vi "Read UDP Data.vi"(8 "error in (no error)":errorcluster, 11 "UDP Cluster in":T2) -> (0 "error out":errorcluster, 3 "UDP Cluster out":T2)   [LabVIEW 2013, in "Workspace MultiY Graph.lvlib"]
uses:
  Workspace MultiY Graph.lvlib
  UDP Stream Configuration.ctl
  <vilib>/NI Veristand/Execution/Workspace/UDP Stream Packet.ctl
  <vilib>/NI Veristand/Execution/Workspace/NI_VS Workspace ExecutionAPI.lvlib
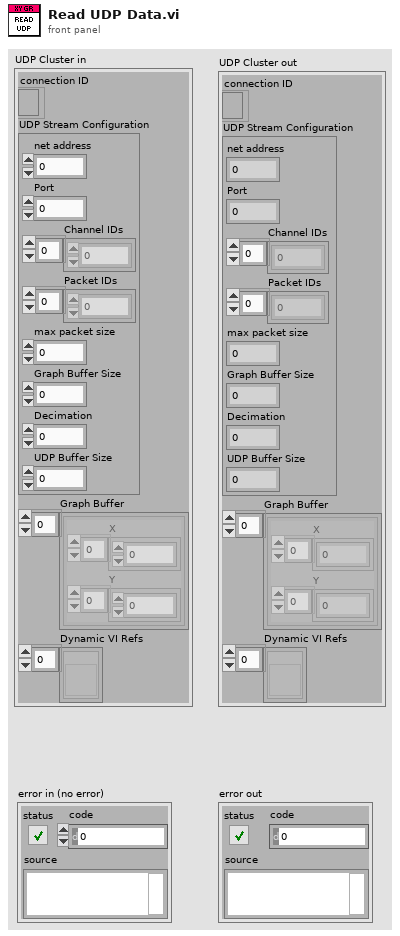
[diagram p1: front panel]
types:
  T1 = typedef "Workspace MultiY Graph.lvlib/UDP Stream Configuration.ctl" = cluster{"net address":u32, "Port":u16, "Channel IDs":i32[], "Packet IDs":i32[], "max packet size":i32, "Graph Buffer Size":i32, "Decimation":i32, "UDP Buffer Size":u32}
  T2 = cluster{"connection ID":refnum<k16>, "UDP Stream Configuration":T1, "Graph Buffer":cluster{"X":dbl[], "Y":dbl[]}[], "Dynamic VI Refs":refnum<vi>[]}
  T3 = typedef "NI_VS Workspace ExecutionAPI.lvlib/UDP Stream Packet.ctl" = cluster{"ID":i32, "t0":dbl, "dt":dbl, "Channel IDs":i32[], "Channel Data":dbl[][], "Sample Offset":u64}
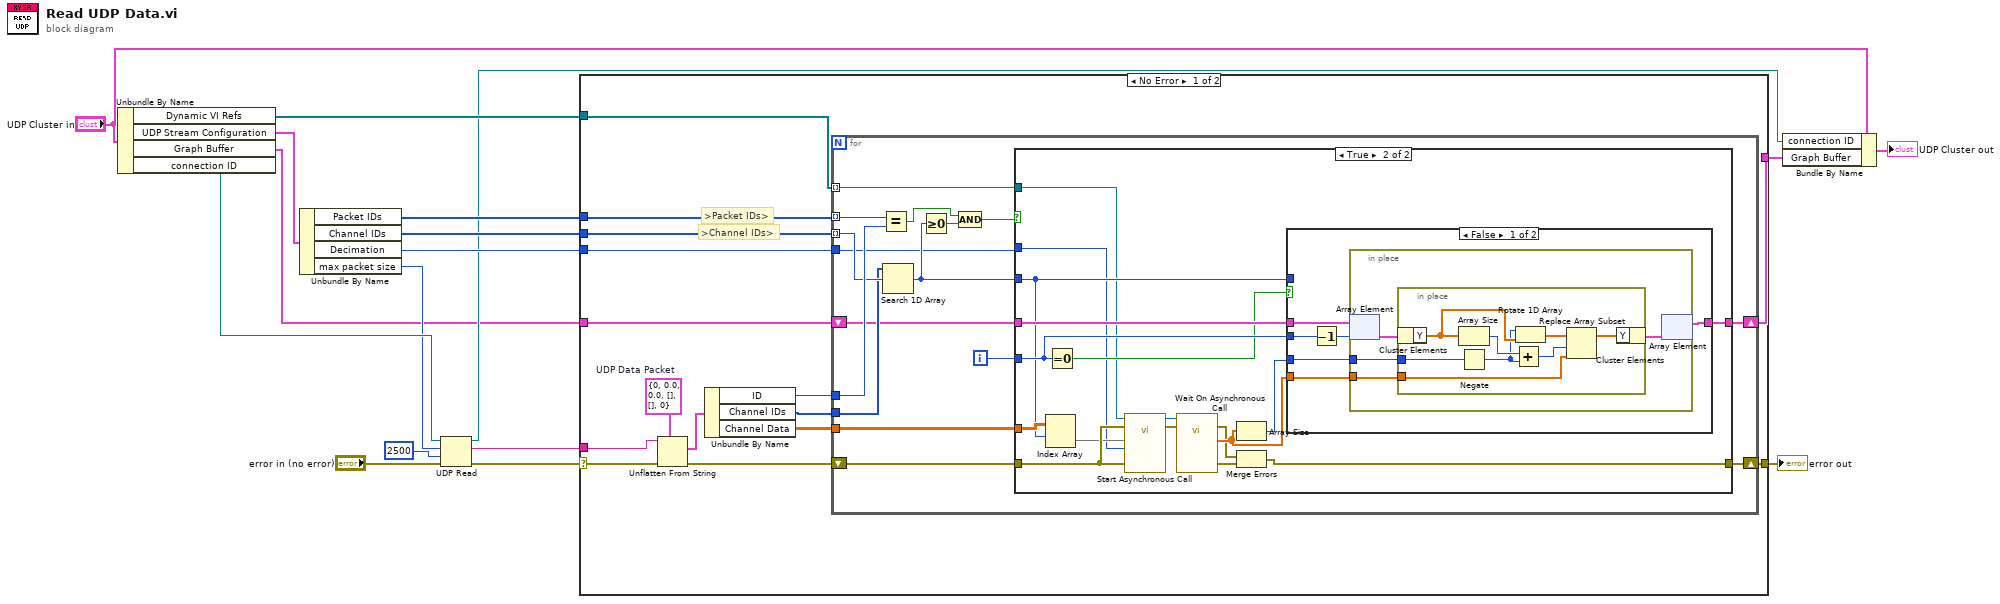
[diagram p0: block diagram]
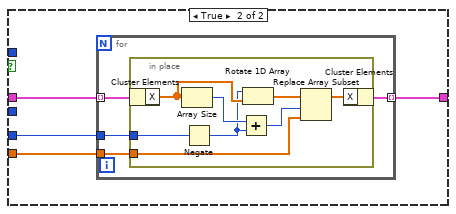
[diagram p3: hidden frame]
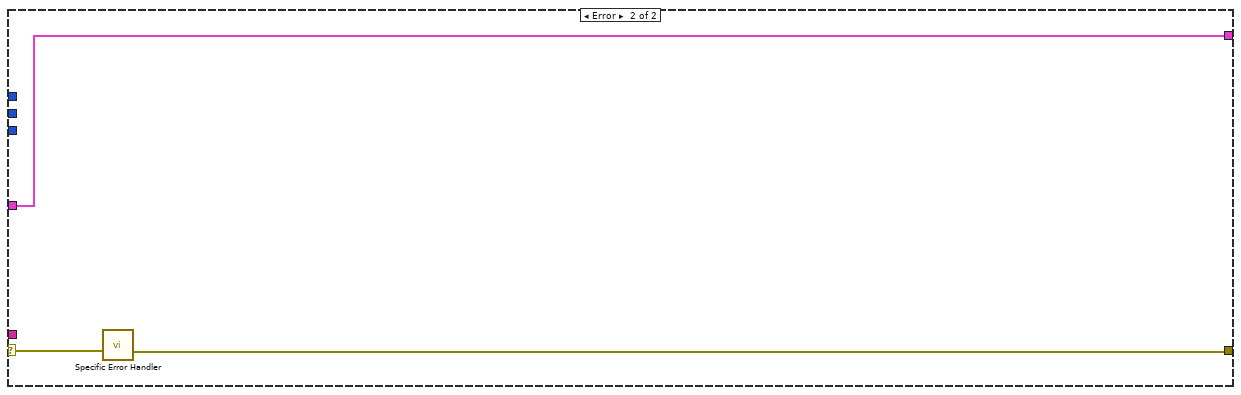
[diagram p4: hidden frame]
diagram:
  n1 = Unbundle By Name("UDP Cluster in") -> ("Dynamic VI Refs"=w10:refnum<vi>[], "UDP Stream Configuration"=w6:T1, "Graph Buffer"=w3:cluster{"X":dbl[], "Y":dbl[]}[], "connection ID"=w5:refnum<k16>)
  n2 = Unbundle By Name(w6) -> ("Packet IDs"=w13:i32[], "Channel IDs"=w17:i32[], "Decimation"=w12:i32, "max packet size"=w4:i32)
  n3 = UDP Read(connection ID=w5, max size (548)=w4, timeout ms (25000)=2500, 8:"error in (no error)") -> (data out=w15:string, error out=w2:errorcluster, 3:w9:refnum<k16>)  [unwired: 2 out]
  n4 = case shown="No Error" w2 {
    selector: w2 -> [w18 w104]
    tunnel: w17 -> [w32 _]
    tunnel: w15 -> [w27 _]
    tunnel: w13 -> [w25 _]
    tunnel: w12 -> [w24 _]
    tunnel: [w22 w103] -> w11
    tunnel: w10 -> [w21 _]
    tunnel: [w20 w102] -> w8
    tunnel: w3 -> [w19 w102]
    frame No Error {
      w26 = T3 {"ID"=0, "t0"=0.0, "dt"=0.0, "Channel IDs"=[], "Channel Data"=[], "Sample Offset"=0}  # UDP Data Packet
      # ">Packet IDs>"
      # ">Channel IDs>"
      n5 = Unflatten From String(type=w26, binary string=w27, error in (no error)=w18) -> (value=w31:T3, error out=w23:errorcluster)  [unwired: 2 in, 1 out]
      n6 = Unbundle By Name(w31) -> ("ID"=w28:i32, "Channel IDs"=w29:i32[], "Channel Data"=w30:dbl[][])
      n7 = for {
        tunnel: w32 -> [w46] mode=indexing
        tunnel: w25 -> [w48] mode=indexing
        tunnel: w28 -> [w47]
        tunnel: w30 -> [w40]
        tunnel: w29 -> [w39]
        shift-right: [w37] -> w20
        shift-left: w19 -> [w38]
        tunnel: w21 -> [w36] mode=indexing
        tunnel: w24 -> [w35]
        shift-right: [w33] -> w22
        shift-left: w23 -> [w34]
        i -> [w41]
        n8 = Equal?(x=w48, y=w47) -> (x = y?=w45:bool)
        n9 = Search 1D Array(1D array=w39, element=w46) -> (index of element=w42:i32)  [unwired: 1 in]
        n10 = Greater Or Equal To 0?(x=w42) -> (x >= 0?=w44:bool)
        n11 = Compound Arithmetic op=AND(w45, w44) -> (w43:bool)
        n12 = case shown="True" w43 {
          tunnel: w42 -> [_ w62]
          tunnel: w41 -> [_ w65]
          tunnel: w40 -> [_ w63]
          tunnel: w38 -> [w50 w67]
          tunnel: [w50 w66] -> w37
          tunnel: w36 -> [_ w60]
          tunnel: w35 -> [_ w56]
          tunnel: w34 -> [w49 w59]
          tunnel: [w49 w58] -> w33
          frame False {
            # "This channel is not in this UDP Data Packet."
          }
          frame True {
            n13 = Index Array(array=w63, index (row)=w62) -> (element=w57:dbl[])  [unwired: 1 in]
            n14 = Equal To 0?(x=w65) -> (x = 0?=w64:bool)
            n15 = call-by-ref "Start Asynchronous Call"(reference=w60, error in=w59, 8:"error in (no error)"=w59, "decimating factor"=w56, "X"=w57) -> (reference out=w55:refnum<vi>, error out=w54:errorcluster)  [unwired: 7 in, 2 out]
            n16 = call-by-ref "Wait On Asynchronous Call"(reference=w55, error in=w54) -> (error out=w51:errorcluster, 0:"error out"=w52:errorcluster, "Decimated Array"=w53:dbl[])  [unwired: 10 in, 1 out]
            n17 = Array Size(array=w53) -> (size(s)=w61:i32)
            n18 = Merge Errors(w51, w52) -> (w58:errorcluster)
            n19 = case shown="False" w64 {
              tunnel: w67 -> [w73 w89]
              tunnel: w62 -> [_ _]
              tunnel: [w72 w88] -> w66
              tunnel: w65 -> [w71 _]
              tunnel: w61 -> [w69 w87]
              tunnel: w53 -> [w68 w86]
              frame False {
                n20 = Decrement(x=w71) -> (x-1=w70:i32)
                n21 = in-place {
                  in-place-border: w69 -> [w75]
                  in-place-border: w68 -> [w74]
                  n22 = in-place-array #1(w73, w70) -> (w77:cluster{"X":dbl[], "Y":dbl[]})
                  n23 = in-place {
                    in-place-border: w75 -> [w85]
                    in-place-border: w74 -> [w78]
                    n24 = in-place-cluster #2(w77) -> ("Y"=w83:dbl[])
                    n25 = Array Size(array=w83) -> (size(s)=w82:i32)
                    n26 = Negate(x=w85) -> (-x=w81:i32)
                    n27 = Add(x=w82, y=w81) -> (x+y=w80:i32)
                    n28 = Rotate 1D Array(1:w83, 2:w81) -> (0:w84:dbl[])
                    n29 = Replace Array Subset(array=w84, new element=w78, index=w80) -> (w79:dbl[])
                    n30 = in-place-cluster #2("Y"=w79) -> (w76:cluster{"X":dbl[], "Y":dbl[]})
                  }
                  n31 = in-place-array #1(w76) -> (w72:cluster{"X":dbl[], "Y":dbl[]}[])  [unwired: 1 out]
                }
              }
              frame True {
                n32 = for {
                  tunnel: w87 -> [w93]
                  tunnel: w89 -> [w91] mode=indexing
                  tunnel: [w92] -> w88 mode=indexing
                  tunnel: w86 -> [w90]
                  n33 = in-place {
                    in-place-border: w93 -> [w101]
                    in-place-border: w90 -> [w94]
                    n34 = in-place-cluster #3(w91) -> ("X"=w99:dbl[])
                    n35 = Array Size(array=w99) -> (size(s)=w98:i32)
                    n36 = Negate(x=w101) -> (-x=w97:i32)
                    n37 = Add(x=w98, y=w97) -> (x+y=w96:i32)
                    n38 = Rotate 1D Array(1:w99, 2:w97) -> (0:w100:dbl[])
                    n39 = Replace Array Subset(array=w100, new element=w94, index=w96) -> (w95:dbl[])
                    n40 = in-place-cluster #3("X"=w95) -> (w92:cluster{"X":dbl[], "Y":dbl[]})
                  }
                }
              }
            }
          }
        }
      }
    }
    frame Error {
      n41 = call "Specific Error Handler"("Error to Check"=w104) -> ("error out"=w103:errorcluster)  [unwired: 11 in, 3 out]
    }
  }
  "error out" <- w11
  n42 = Bundle By Name(cluster="UDP Cluster in", "connection ID"=w9, "Graph Buffer"=w8) -> (→"UDP Cluster out":T2)
